vi "Reset INT.vi"(8 "error in (no error)":errorcluster, 11 "CAP1208 in":refnum<class "CAP1208.lvclass">) -> (0 "error out":errorcluster, 3 "CAP1208 out":refnum<class "CAP1208.lvclass">)   [LabVIEW 2020, in "CAP1208.lvclass"]
uses:
  CAP1208.lvclass
  CAP1208.lvclass/CAP1208.ctl
  Read I2C.vi
  Write I2C.vi
  LINX I2C/LINX I2C.lvclass
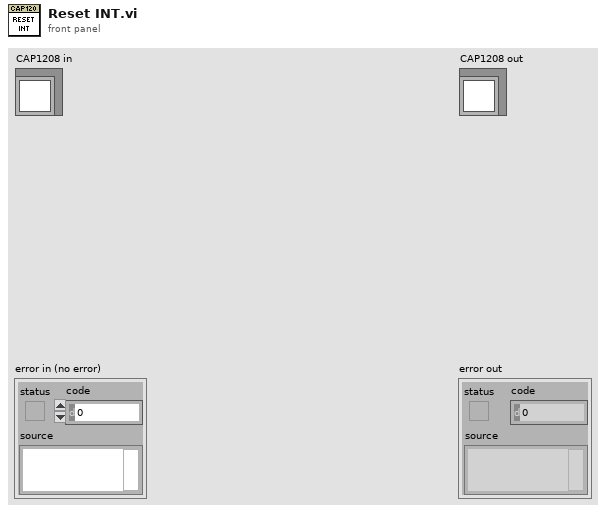
[diagram p1: front panel]
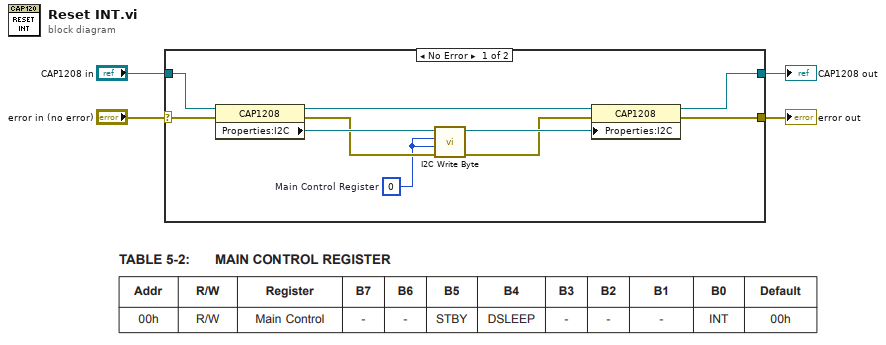
[diagram p0: block diagram]
diagram:
  n1 = case shown="No Error" "error in (no error)" {
    selector: "error in (no error)" -> [w10 w16]
    tunnel: [w13 w16] -> w3
    tunnel: [w12 w15] -> w1
    tunnel: "CAP1208 in" -> [w14 w15]
    frame No Error {
      w5 = u8 0  # Main Control Register
      n2 = property class="CAP1208"(reference=w14, error in=w10) -> (reference out=w11:refnum<class "CAP1208.lvclass">, error out=w8:errorcluster, "Properties:I2C"=w9:refnum<class "LINX I2C.lvclass">)
      n3 = call "I2C Write Byte.vi"("error in (no error)"=w8, "Value"=w5, "Register Address"=w5, "LINX I2C in"=w9) -> ("error out"=w6:errorcluster, "LINX I2C out"=w7:refnum<class "LINX I2C.lvclass">)  [unwired: 6 in]
      n4 = property class="CAP1208"(reference=w11, error in=w6, "Properties:I2C"=w7) -> (reference out=w12:refnum<class "CAP1208.lvclass">, error out=w13:errorcluster)
    }
    frame Error {
    }
  }
  "error out" <- w3
  "CAP1208 out" <- w1
